vi "4Pi 4Pi Modes - Fit Sum ROIs.vi"(2 "Blink Analysis Type":T1=1 items=["Mean Intensity", "2D Fit Intensity"], 7 "ROIs":u16[][][](array[numeric])) -> (8 "Blink Metric":dbl)   [LabVIEW 2016]
uses:
  4Pi 4Pi Modes - Controls/4Pi 4Pi Modes - Mode Scan - Blink Analysis Type.ctl
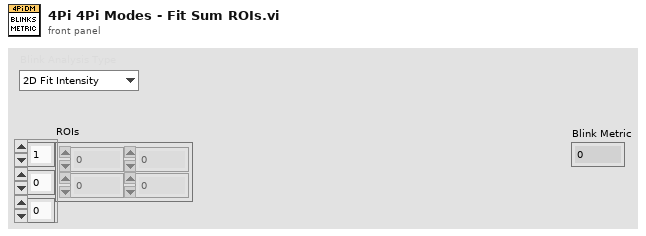
[diagram p1: front panel]
types:
  T1 = typedef "4Pi 4Pi Modes - Mode Scan - Blink Analysis Type.ctl" = u16
  T2 = typedef "2D Gaussian - Best Fit Parameters.ctl" = cluster{"Amplitude":dbl, "X Position":dbl, "Y Position":dbl, "X Width":dbl, "Y Width":dbl, "Offset":dbl}
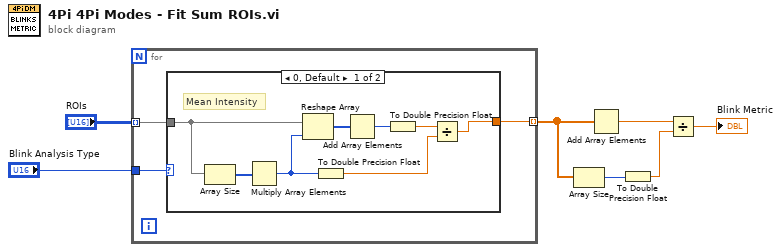
[diagram p0: block diagram]
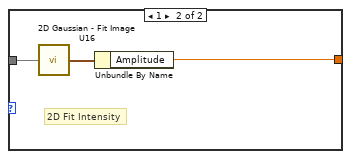
[diagram p2: hidden frame]
diagram:
  n1 = for {
    tunnel: "ROIs" -> [w10] mode=indexing
    tunnel: [w9] -> w5 mode=indexing
    tunnel: "Blink Analysis Type" -> [w8]
    n2 = case shown="0, Default" w8 {
      tunnel: w10 -> [w18 w21]
      tunnel: [w11 w19] -> w9
      frame 0, Default {
        # "Mean Intensity"
        n3 = Array Size(array=w18) -> (size(s)=w17:i32[])
        n4 = Multiply Array Elements(1:w17) -> (0:w14:i32)
        n5 = Reshape Array(w18, w14) -> (w16:u16[])
        n6 = To Double Precision Float(number=w14) -> (double precision float=w12:dbl)
        n7 = Add Array Elements(numeric array=w16) -> (sum=w15:u16)
        n8 = To Double Precision Float(number=w15) -> (double precision float=w13:dbl)
        n9 = Divide(x=w13, y=w12) -> (x/y=w11:dbl)
      }
      frame 1 {
        # "2D Fit Intensity"
        n10 = call "2D Gaussian - Fit Image U16.vi"("Image In (U16)"=w21) -> ("Best Fit Params"=w20:T2)  [unwired: 13 in, 1 out]
        n11 = Unbundle By Name(w20) -> ("Amplitude"=w19:dbl)
      }
    }
  }
  n12 = Array Size(array=w5) -> (size(s)=w4:i32)
  n13 = Add Array Elements(numeric array=w5) -> (sum=w3:dbl)
  n14 = To Double Precision Float(number=w4) -> (double precision float=w2:dbl)
  n15 = Divide(x=w3, y=w2) -> (x/y=→"Blink Metric":dbl)
